vi "ThreePts_RotationMatrix.vi"(2 "Circumcenter":dbl[](array[numeric]), 3 "V 2":dbl[](array[numeric]), 4 "V 1":dbl[](array[numeric])) -> (0 "Circumcenter":dbl[](array[numeric]), 1 "Rotation Matrix ( Local to Global )":dbl[][](array[numeric]))   [LabVIEW 2012, in "Force Field Controller.lvclass"]
uses:
  Force Field Controller.lvclass
  <vilib>/Analysis/NI_AALPro.lvlib
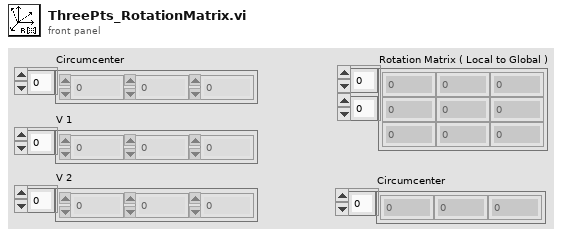
[diagram p1: front panel]
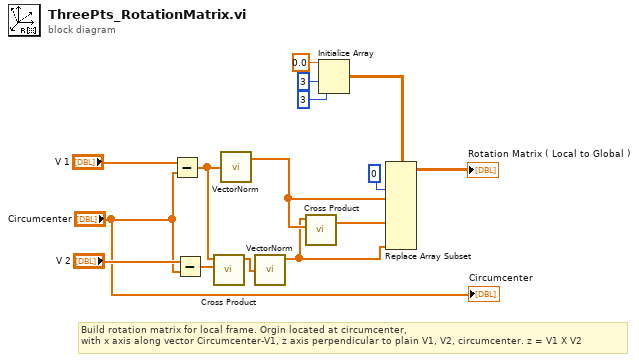
[diagram p0: block diagram]
diagram:
  # "Build rotation matrix for local frame. Orgin located at circumcenter, \nwith x axis along vector Circumcenter-V1, z axis perpendicular to plain V1, V2, circumcenter. z = V1 X V2"
  n1 = Subtract(x="V 1", y="Circumcenter") -> (x-y=w4:dbl[])
  n2 = Subtract(x="V 2", y="Circumcenter") -> (x-y=w8:dbl[])
  n3 = call <vilib>:"Cross Product.vi"("B Vector"=w8, "A Vector"=w4) -> ("Cross Product"=w2:dbl[])  [unwired: 8 in, 1 out]
  n4 = call "VectorNorm.vi"("Vector"=w4) -> ("Unit Vector"=w3:dbl[])  [unwired: 1 out]
  n5 = call "VectorNorm.vi"("Vector"=w2) -> ("Unit Vector"=w1:dbl[])  [unwired: 1 out]
  n6 = call <vilib>:"Cross Product.vi"("B Vector"=w3, "A Vector"=w1) -> ("Cross Product"=w9:dbl[])  [unwired: 8 in, 1 out]
  n7 = Initialize Array(0.0 ("element"), 3 ("dimension size"), 3 ("dimension size")) -> (w11:dbl[][])
  n8 = Replace Array Subset(array=w11, new element #1=w3, index (col) #1=0 ("disabled index (col)"), new element #2=w9, new element #3=w1) -> (→"Rotation Matrix ( Local to Global )":dbl[][])  [unwired: 5 in]
  "Circumcenter" <- "Circumcenter"
